vi "Live window-Refresh graphs.vi"(5 "Grid Lines":u32=2 min=2 max=10 step=1, 7 "Visible(Grid)":bool, 9 "Right Channel":T2, 10 "Left Channel":T2, 11 "Element to queue":T3) -> (0 "Right image":T1, 1 "Enable right image":bool, 2 "Enable left image":bool, 3 "Left image":T1)   [LabVIEW 2017]
uses:
  Queue/Live graphs queue/Typedefs/Live imaging queue element.ctl
  <vilib>/vision/Image Controls.llb/IMAQ Image.ctl
  Typedefs/Channel Selector.ctl
  Typedefs/Left-Right enum.ctl
  Global Variables/gl_UI Ctrl Refs.vi
panel:
  out "error out 2":errorcluster
  out "error out":errorcluster
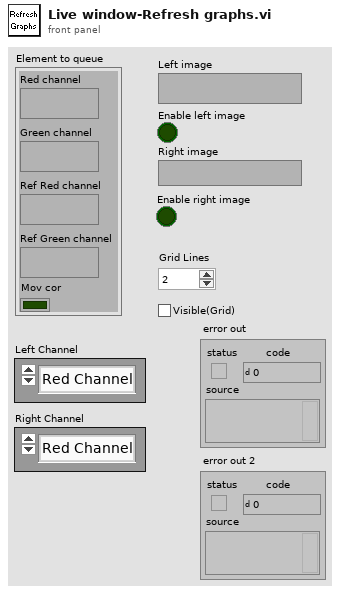
[diagram p1: front panel]
types:
  T1 = typedef "IMAQ Image.ctl" = refnum<image>
  T2 = typedef "Channel Selector.ctl" = enum16{"Red Channel", "Green Channel", "Blended"}
  T3 = typedef "Live imaging queue element.ctl" = cluster{"Red channel":T1, "Green channel":T1, "Ref Red channel":T1, "Ref Green channel":T1, "Mov cor":bool}
  T4 = typedef "Left-Right enum.ctl" = enum16{"Right", "Left"}
  T5 = typedef "UI ctrl refs cluster.ctl" = cluster{"Top level VI path":path, "Top level VI ref":refnum<vi>, "User menu ref":refnum<k9>, "Sub Panel control":refnum<vi>, "Imaging Param Tab":refnum<vi>, "Occurrence-Start drivers":refnum<k4>, "Occurrence-Speed logging initialised":refnum<k4>, "Occurrence-XYZ stage initialised":refnum<k4>, "Exit button":refnum<vi>, "Status ind":refnum<vi>, "Set as origin":refnum<vi>, "Speed Logging":refnum<vi>, "Time Lapse":refnum<vi>, "Live Imaging":refnum<vi>, "AOL Z Stack":refnum<vi>, "Motor Z Stack":refnum<vi>, "Funct Acq button":refnum<vi>, "Hard Shutter":refnum<vi>, "Virtual Shutter":refnum<vi>, "Laser Power":refnum<vi>, "AOL Mode":refnum<vi>, "Frame Size":refnum<vi>, "Field of View":refnum<vi>, "Dwell Time":refnum<vi>, "Zoom":refnum<vi>, "AOL Z":refnum<vi>, "Objective":refnum<vi>, "Axis":refnum<vi>, "Paths & Names":refnum<vi>, "Experiment folder path (ind.)":refnum<vi>, "Last State (Ind.)":refnum<vi>, "Averages":refnum<vi>, "Angle (degrees)":refnum<vi>, "X centre":refnum<vi>, "Y centre":refnum<vi>, "Plane Mode":refnum<vi>, "# Planes":refnum<vi>, "Z Start":refnum<vi>, "Z Stop":refnum<vi>, "Z Step":refnum<vi>, "PMT 1":refnum<vi>, "PMT 2":refnum<vi>, "Stage XYZ Position":refnum<vi>, "Pockels@Z Start":refnum<vi>, "Pockels@Z Stop":refnum<vi>, "Obtain Z Start":refnum<vi>, "Obtain Z Stop":refnum<vi>, "Live stim.trig.period":refnum<vi>, "Live stim.trig.enable":refnum<vi>, "Movement Correction":refnum<vi>, "Load Reference Image":refnum<vi>, "XY Stage Move":refnum<vi>, "MovCor Cluster":refnum<vi>, "RefDAQParam":refnum<vi>, "Funct. Acq. Pockels Modulation":refnum<vi>, "Ref Laser Power":refnum<vi>, "Enable Video Recording":refnum<vi>, "Video Record-Live Imaging":refnum<vi>, "Video Record-Funct acq":refnum<vi>, "Reference Source":refnum<vi>, "AOL Z-stack Chirps Ready (ind)":refnum<vi>, "Target time between mov.cor. ref triggers (ms)":refnum<vi>, "Funct. Acq. Ref frame save":refnum<vi>, "Tracking button":refnum<vi>, "Show ref plots window":refnum<vi>, "Center freq ind (nm)":refnum<vi>, "Pickup mode (ind)":refnum<vi>, "Logging queue (ind)":refnum<vi>, "Back aperture power (ind.)":refnum<vi>, "Power after objective (ind.)":refnum<vi>, "Switch user":refnum<vi>, "Ls1 Conn. Status":refnum<vi>, "Ls1Tuning Status":refnum<vi>, "Ls1 Faults":refnum<vi>, "Ls1 Connection":refnum<vi>, "Ls1 Mode":refnum<vi>, "Ls1 POWER [mW]":refnum<vi>, "Ls1Shutter":refnum<vi>, "Ls1 Wavelength":refnum<vi>, "Ls1 Note":refnum<vi>, "Ls1 Confirm Wav":refnum<vi>, "Ls1 PreChrp Prism1":refnum<vi>, "Ls1 PreChrp Prism2":refnum<vi>, "Ls1 wav top Ind":refnum<vi>, "Ls1 power top Ind":refnum<vi>, "Ls1 Pump peak Hold":refnum<vi>, "Ls1 Status Ind":refnum<vi>, "Ls1 wav cancel":refnum<vi>, "Experiment Type":refnum<vi>, "Biology Information":refnum<vi>}
  T6 = typedef "PMT control knob.ctl" = u16
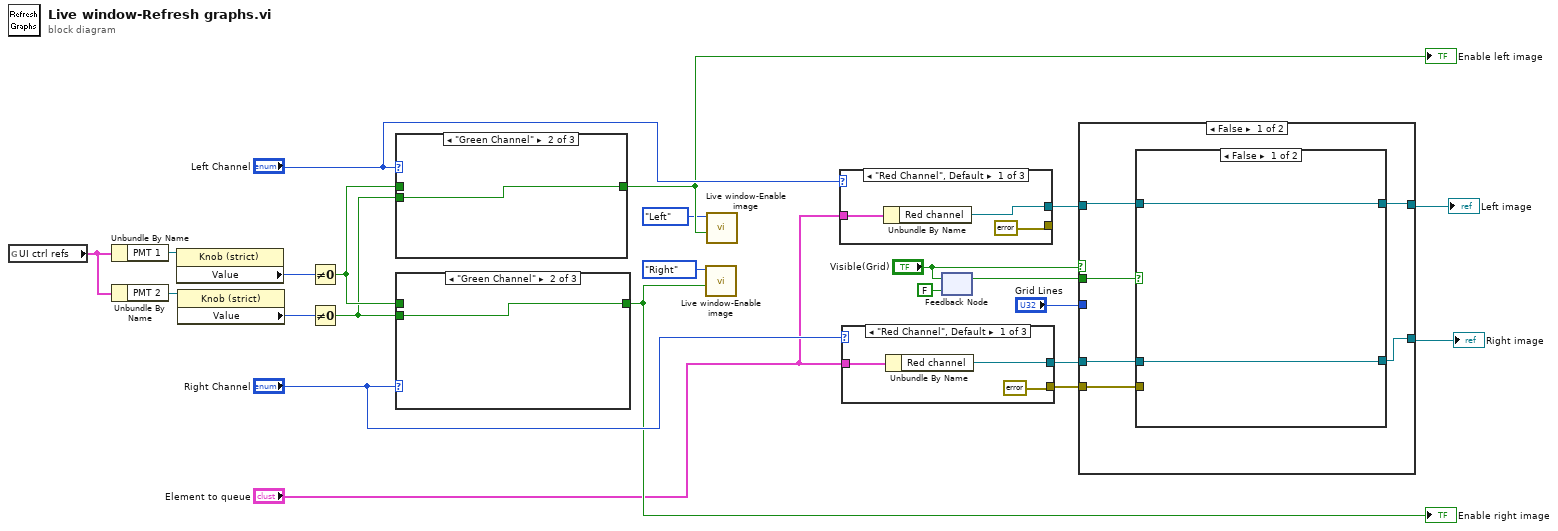
[diagram p0: block diagram]
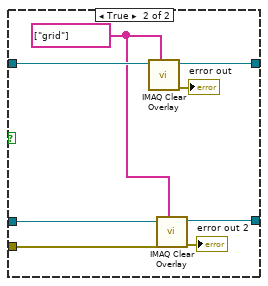
[diagram p2: hidden frame]
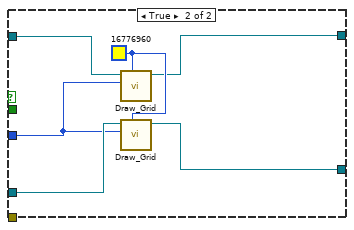
[diagram p3: hidden frame]
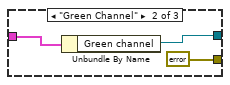
[diagram p4: hidden frame]
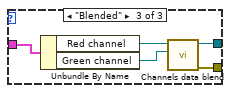
[diagram p5: hidden frame]
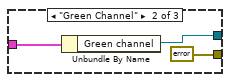
[diagram p6: hidden frame]
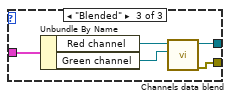
[diagram p7: hidden frame]
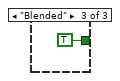
[diagram p9: hidden frame]
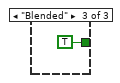
[diagram p11: hidden frame]
diagram:
  n1 = global read "gl_UI Ctrl Refs.vi" "UI ctrl refs"() -> (w19:T5)
  n2 = Unbundle By Name(w19) -> ("PMT 1"=w21:refnum<vi>)
  n3 = Unbundle By Name(w19) -> ("PMT 2"=w20:refnum<vi>)
  n4 = property on="Property Node" class="Knob (strict)"(reference=w21) -> ("Value"=w18:T6)  [unwired: 1 in, 2 out]
  n5 = property on="Property Node" class="Knob (strict)"(reference=w20) -> ("Value"=w17:T6)  [unwired: 1 in, 2 out]
  n6 = Not Equal To 0?(x=w18) -> (x != 0?=w13:bool)
  n7 = Not Equal To 0?(x=w17) -> (x != 0?=w12:bool)
  n8 = case shown="\"Green Channel\"" "Left Channel" {
    tunnel: w13 -> [w24 _ _]
    tunnel: w12 -> [_ w25 _]
    tunnel: [w24 w25 TRUE] -> w16
    frame "Red Channel", Default {
    }
    frame "Green Channel" {
    }
    frame "Blended" {
    }
  }
  "Enable left image" <- w16
  n9 = case shown="\"Green Channel\"" "Right Channel" {
    tunnel: w13 -> [w27 _ _]
    tunnel: w12 -> [_ w28 _]
    tunnel: [w27 w28 TRUE] -> w15
    frame "Red Channel", Default {
    }
    frame "Green Channel" {
    }
    frame "Blended" {
    }
  }
  "Enable right image" <- w15
  n10 = call "Live window-Enable image.vi"("Enable"=w15, "Which image display?"=Left-Right_enum."Right") -> ()  [unwired: 10 in]
  n11 = call "Live window-Enable image.vi"("Enable"=w16, "Which image display?"=Left-Right_enum."Left") -> ()  [unwired: 10 in]
  n12 = case shown="\"Red Channel\", Default" "Left Channel" {
    tunnel: "Element to queue" -> [w32 w35 w40]
    tunnel: [w31 w34 w37] -> w9
    tunnel: [errorcluster {"status"=FALSE, "code"=0, "source"=""} ("error out") errorcluster {"status"=FALSE, "code"=0, "source"=""} ("error out") w36] -> _
    frame "Red Channel", Default {
      n13 = Unbundle By Name(w32) -> ("Red channel"=w31:T1)
    }
    frame "Green Channel" {
      n14 = Unbundle By Name(w35) -> ("Green channel"=w34:T1)
    }
    frame "Blended" {
      n15 = Unbundle By Name(w40) -> ("Red channel"=w39:T1, "Green channel"=w38:T1)
      n16 = call "Channels data blend.vi"("GREEN"=w38, "RED"=w39) -> ("error out"=w36:errorcluster, "Image Out"=w37:T1)  [unwired: 8 in]
    }
  }
  n17 = case shown="\"Red Channel\", Default" "Right Channel" {
    tunnel: "Element to queue" -> [w43 w46 w51]
    tunnel: [w42 w45 w48] -> w8
    tunnel: [errorcluster {"status"=FALSE, "code"=0, "source"=""} ("error out") errorcluster {"status"=FALSE, "code"=0, "source"=""} ("error out") w47] -> w4
    frame "Red Channel", Default {
      n18 = Unbundle By Name(w43) -> ("Red channel"=w42:T1)
    }
    frame "Green Channel" {
      n19 = Unbundle By Name(w46) -> ("Green channel"=w45:T1)
    }
    frame "Blended" {
      n20 = Unbundle By Name(w51) -> ("Red channel"=w50:T1, "Green channel"=w49:T1)
      n21 = call "Channels data blend.vi"("GREEN"=w49, "RED"=w50) -> ("error out"=w47:errorcluster, "Image Out"=w48:T1)  [unwired: 8 in]
    }
  }
  n22 = feedback-in #1("Visible(Grid)") -> ()
  n23 = feedback #1(FALSE ("Visible(Grid)")) -> (w1:bool)
  n24 = case shown="False" "Visible(Grid)" {
    tunnel: w9 -> [w57 w72]
    tunnel: w8 -> [w56 w71]
    tunnel: [w54 w70] -> w7
    tunnel: [w53 w69] -> w6
    tunnel: "Grid Lines" -> [_ w68]
    tunnel: w4 -> [w55 _]
    tunnel: w1 -> [w52 _]
    frame False {
      n25 = case shown="False" w52 {
        tunnel: w57 -> [w59 w67]
        tunnel: w56 -> [w58 w66]
        tunnel: w55 -> [_ w64]
        tunnel: [w59 w63] -> w54
        tunnel: [w58 w62] -> w53
        frame False {
        }
        frame True {
          w65 = string[] ["grid"] ("Groups")
          n26 = call "IMAQ Clear Overlay"("Groups"=w65, "Image"=w67) -> ("error out"=→"error out":errorcluster, "Image Out"=w63:T1)  [unwired: 8 in]
          n27 = call "IMAQ Clear Overlay"("Groups"=w65, "error in (no error)"=w64, "Image"=w66) -> ("error out"=→"error out 2":errorcluster, "Image Out"=w62:T1)  [unwired: 7 in]
        }
      }
    }
    frame True {
      w73 = u32 16776960
      n28 = call "Draw_Grid.vi"("Grid Line Color"=w73, "Grid Lines"=w68, "Image In"=w72) -> ("Image Out"=w70:T1)  [unwired: 7 in, 1 out]
      n29 = call "Draw_Grid.vi"("Grid Line Color"=w73, "Grid Lines"=w68, "Image In"=w71) -> ("Image Out"=w69:T1)  [unwired: 7 in, 1 out]
    }
  }
  "Left image" <- w7
  "Right image" <- w6
